vi "ProgressBar.vi"(1 "stop":bool, 2 "String":string, 3 "MaxRange":i32) -> ()   [LabVIEW 2013]
panel:
  in  "abort":bool
  out "Slide":i32(slide) scale=0.0..2285.0
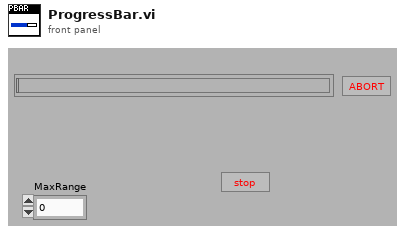
[diagram p1: front panel]
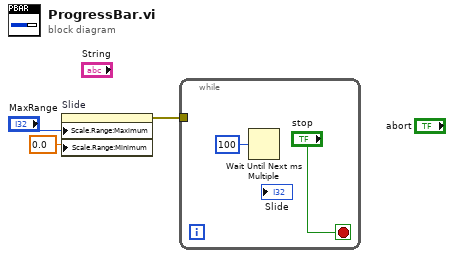
[diagram p0: block diagram]
diagram:
  n1 = property on="Slide" class="Slide (strict)"("Scale.Range:Maximum"="MaxRange", "Scale.Range:Minimum"=0.0) -> (error out=w1:errorcluster)  [unwired: 2 in, 1 out]
  n2 = while {
    tunnel: w1 -> [_]
    stop <- "stop" stop-if-true
    n3 = Wait Until Next ms Multiple(millisecond multiple=u32 100) -> ()  [unwired: 1 out]
  }
